vi "start.vi"(8 "error in (no error)":errorcluster, 11 "NetworkPixelfly in":refnum<class "NetworkPixelfly.lvclass">) -> (0 "error out":errorcluster, 3 "NetworkPixelfly out":refnum<class "NetworkPixelfly.lvclass">)   [LabVIEW 2011, in "Hardware.lvlib" / "HWControllers.lvlib" / "NetworkPixelfly.lvclass"]
uses:
  NetworkPixelfly.lvclass
  NetworkPixelfly.lvclass/NetworkPixelfly.ctl
  Channels/Camera/PixelflySA/PixelflySA.lvclass
  Channels/Channels.lvlib
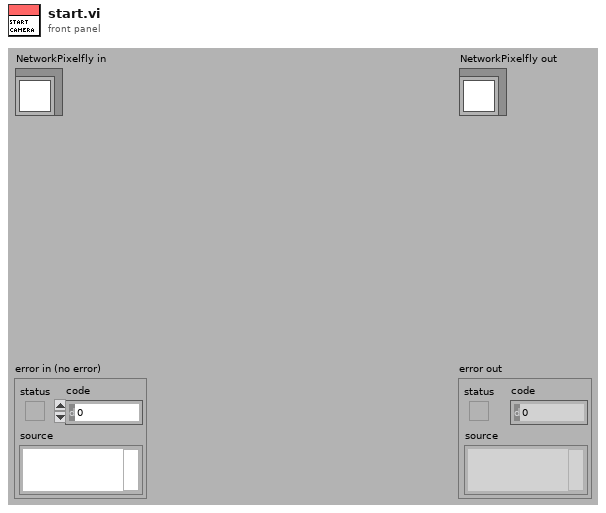
[diagram p1: front panel]
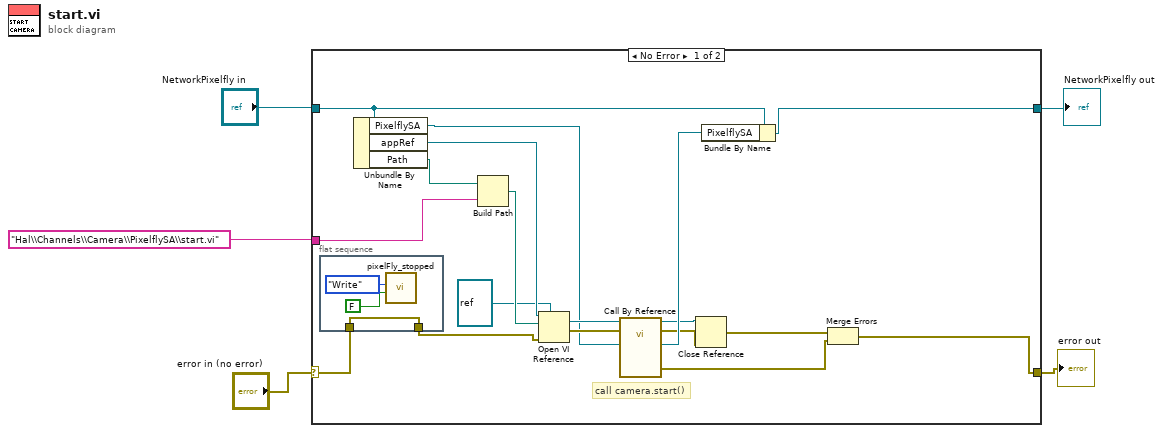
[diagram p0: block diagram]
diagram:
  n1 = case shown="No Error" "error in (no error)" {
    selector: "error in (no error)" -> [w7 w28]
    tunnel: [w9 w28] -> w2
    tunnel: [w8 w27] -> w1
    tunnel: "NetworkPixelfly in" -> [w15 w27]
    tunnel: "Hal\\Channels\\Camera\\PixelflySA\\start.vi" ("viPath") -> [w22 _]
    frame No Error {
      # "call camera.start()"
      n2 = flat-sequence {
        tunnel: w7 -> [w24]
        tunnel: [w24] -> w6
        frame #0 {
          n3 = call "pixelFly_stopped.vi"("stop"=FALSE, "Action"=enum16{"Write", "Read"}."Write") -> ()  [unwired: 9 in, 1 out]
        }
      }
      n4 = Unbundle By Name(w15) -> ("PixelflySA"=w16:refnum<class "PixelflySA.lvclass">, "appRef"=w20:refnum<vi>, "Path"=w21:path)
      n5 = Build Path(base path=w21, name or relative path=w22) -> (appended path=w23:path)
      n6 = Open VI Reference(type specifier VI Refnum (for type only)=refnum<vi> refnum, application reference (local)=w20, vi path=w23, error in (no error)=w6) -> (vi reference=w18:refnum<vi>, error out=w17:errorcluster)  [unwired: 2 in]
      n7 = call-by-ref "?"(reference=w18, error in=w17, "Pixelfly in"=w16) -> (reference out=w13:refnum<vi>, error out=w12:errorcluster, 0:"error out"=w11:errorcluster, "Pixelfly out"=w14:refnum<class "PixelflySA.lvclass">)  [unwired: 9 in]
      n8 = Close Reference(reference=w13, error in (no error)=w12) -> (error out=w10:errorcluster)
      n9 = Bundle By Name(cluster=w15, "PixelflySA"=w14) -> (w8:refnum<class "NetworkPixelfly.lvclass">)
      n10 = Merge Errors(w10, w11) -> (w9:errorcluster)
    }
    frame Error {
    }
  }
  "error out" <- w2
  "NetworkPixelfly out" <- w1
